vi "DIO Tasks.vi"(8 "error in":errorcluster, 11 "DIO Cluster":T1) -> (0 "error out":errorcluster)   [LabVIEW 2013]
doc: "Starts a DIO Task for each channel specified in DIO cluster and writes on/off value to the channel"
uses:
  Controls/DIOTypedef.ctl
  <vilib>/DAQmx/write.llb/DAQmx Write (Digital Bool 1Line 1Point).vi
  <vilib>/DAQmx/create/channels.llb/DAQmx Create Channel (DO-Digital Output).vi
  <vilib>/DAQmx/miscellaneous.llb/DAQmx Fill In Error Info.vi
panel:
  # "On/Off      Channel                     Name"
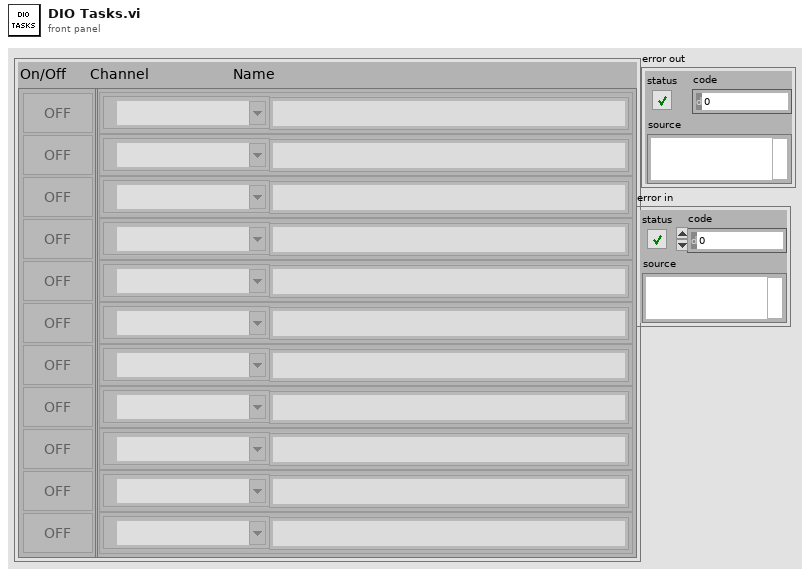
[diagram p1: front panel]
types:
  T1 = typedef "DIOTypedef.ctl" = cluster{"DIO Booleans":bool[], "DIO Channel Array":cluster{"Channel Name":string, "DIO lines":tag}[]}
  T2 = cluster{"Channel Name":string, "DIO lines":tag}[]
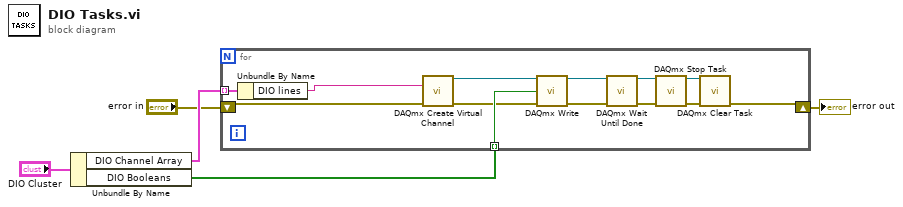
[diagram p0: block diagram]
diagram:
  n1 = Unbundle By Name("DIO Cluster") -> ("DIO Channel Array"=w4:T2, "DIO Booleans"=w3:bool[])
  n2 = for {
    tunnel: w4 -> [w18] mode=indexing
    tunnel: w3 -> [w14] mode=indexing
    shift-right: [w8] -> w2
    shift-left: "error in" -> [w6]
    n3 = Unbundle By Name(w18) -> ("DIO lines"=w13:tag)
    n4 = call-poly <vilib>:"DAQmx Create Virtual Channel.vi"("lines"=w13, "error in"=w6) -> ("task out"=w15:refnum<k21>, "error out"=w7:errorcluster)  [unwired: 12 in]
    n5 = call-poly <vilib>:"DAQmx Write.vi"("task/channels in"=w15, "data"=w14, "error in"=w7) -> ("task out"=w17:refnum<k21>, "error out"=w16:errorcluster)  [unwired: 1 in, 10 out]
    n6 = call <vilib>:"DAQmx Wait Until Done.vi"("task/channels in"=w17, "error in"=w16) -> ("task out"=w10:refnum<k21>, "error out"=w9:errorcluster)  [unwired: 1 in, 11 out]
    n7 = call <vilib>:"DAQmx Stop Task.vi"("task/channels in"=w10, "error in"=w9) -> ("task out"=w12:refnum<k21>, "error out"=w11:errorcluster)  [unwired: 12 in]
    n8 = call <vilib>:"DAQmx Clear Task.vi"("task in"=w12, "error in"=w11) -> ("error out"=w8:errorcluster)  [unwired: 13 in]
  }
  "error out" <- w2
